vi "Update.vi"(8 "error in (no error)":errorcluster, 11 "Timed Loop Controller in":refnum<class "Timed Loop Controller.lvclass">) -> (0 "error out":errorcluster, 3 "Timed Loop Controller out":refnum<class "Timed Loop Controller.lvclass">)   [LabVIEW 2012, in "Timed Loop Controller.lvlib" / "Timed Loop Controller.lvclass"]
uses:
  Timed Loop Controller.lvclass
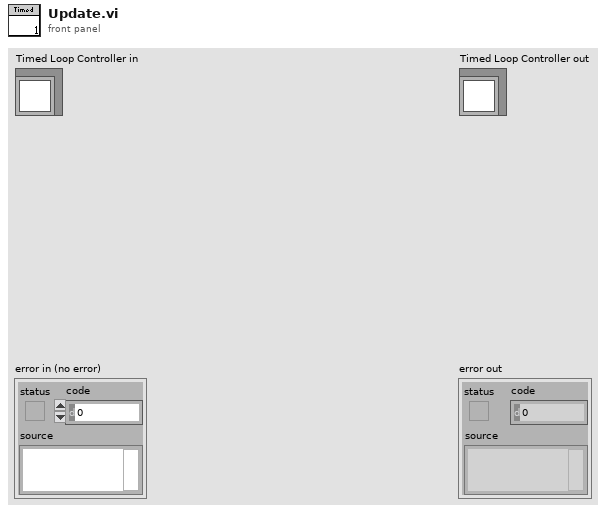
[diagram p1: front panel]
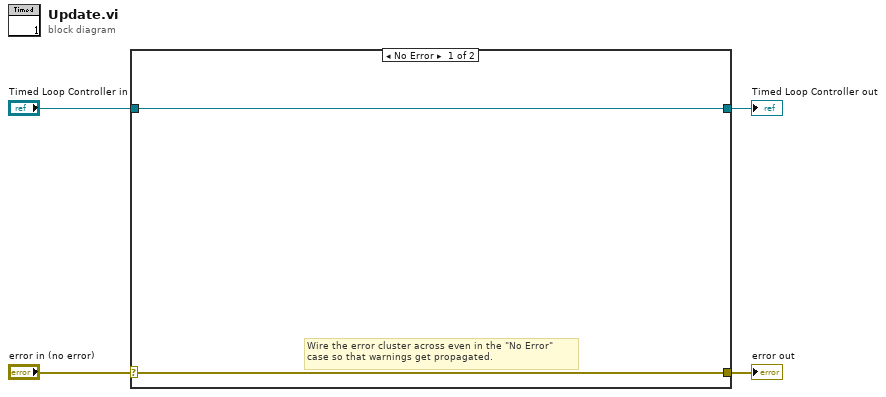
[diagram p0: block diagram]
diagram:
  n1 = case shown="No Error" "error in (no error)" {
    selector: "error in (no error)" -> [w5 w8]
    tunnel: [w5 w8] -> w3
    tunnel: [w6 w7] -> w1
    tunnel: "Timed Loop Controller in" -> [w6 w7]
    frame No Error {
      # "Wire the error cluster across even in the \"No Error\"\ncase so that warnings get propagated."
    }
    frame Error {
    }
  }
  "error out" <- w3
  "Timed Loop Controller out" <- w1
